vi "Increment.vi"(8 "error in":errorcluster, 11 "Increment me":u32=3) -> (0 "error out":errorcluster, 3 "Incremented":u32)   [LabVIEW 2019]
uses:
  target/debug/rust_labview_basic.dll
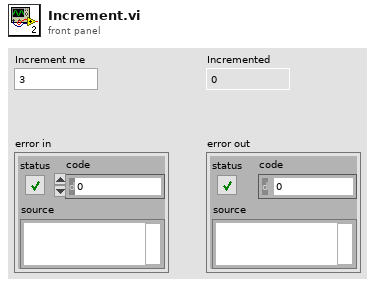
[diagram p1: front panel]
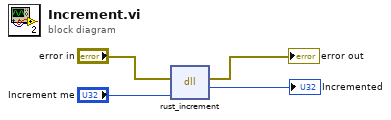
[diagram p0: block diagram]
diagram:
  n1 = dll-call lib="C:/sandbox/rust-labview/rust_labview_basic/target/debug/rust_labview_basic.dll" fn="rust_increment"(error in="error in", "values"="Increment me") -> (error out=→"error out":errorcluster, "return type"=→"Incremented":u32)  [unwired: 3 in, 1 out]
